vi "Read NI 9224.vi"(8 "error in":errorcluster, 11 "NI 9224 in":refnum<class "NI 9224.lvclass">) -> (0 "error out":errorcluster, 1 "channel settings":T1[](array[typedef]), 2 "conversion time":T2, 3 "NI 9224 out":refnum<class "NI 9224.lvclass">)   [LabVIEW 2017, in "Scan Engine Scripting.lvlib" / "NI 9224.lvclass"]
uses:
  NI 9224.lvclass
  Utility/Shared Properties/Conversion Time.ctl
  Mode Classes/Controls/analog channel settings.ctl
  NI 9224.lvclass/NI 9224.ctl
  Scan Engine Scripting.lvlib
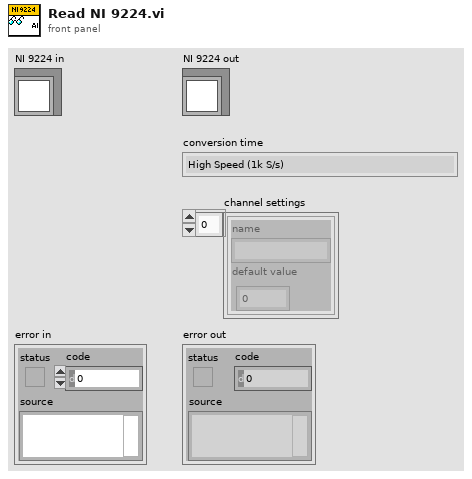
[diagram p1: front panel]
types:
  T1 = typedef "Scan Engine Scripting.lvlib/analog channel settings.ctl" = cluster{"name":string, "default value":dbl}
  T2 = typedef "Scan Engine Scripting.lvlib/Conversion Time.ctl" = enum16{"High Speed (1k S/s)", "Medium Speed (100 S/s)", "Medium Resolution (50/60Hz Rejection - 12 S/s)", "High Resolution (50/60Hz Rejection - 2 S/s)"}
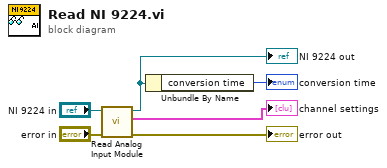
[diagram p0: block diagram]
diagram:
  n1 = call-dynamic "Read Analog Input Module.vi"("error in"="error in", "module in"="NI 9224 in") -> ("error out"=→"error out":errorcluster, "channel settings"=→"channel settings":T1[], "module out"=w2:refnum<class "NI 9224.lvclass">)  [unwired: 7 in]
  "NI 9224 out" <- w2
  n2 = Unbundle By Name(w2) -> ("conversion time"=→"conversion time":T2)
